vi "GUI Init - DIM.vi"(8 "error in (no error)":errorcluster, 9 "Ch.names":string[](array[string]), 10 "Cluster":T1, 11 "Array Ref.":refnum<vi>) -> (0 "error out":errorcluster, 2 "Data":dbl[](array[numeric]), 3 "Array Ref. out":refnum<vi>)   [LabVIEW 2017]
doc: "Initialize array's size and values for DIM Array by reference"
uses:
  Controls/Discrete_GUI_Cluster.ctl
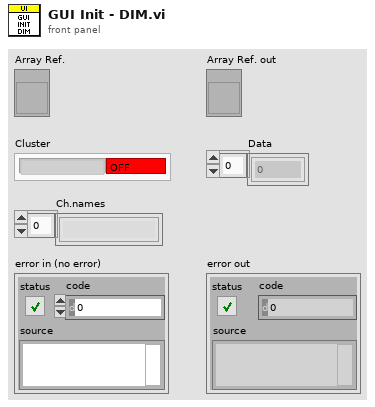
[diagram p1: front panel]
types:
  T1 = typedef "Discrete_GUI_Cluster.ctl" = cluster{"Ch.name":string, "Ch.state":bool}
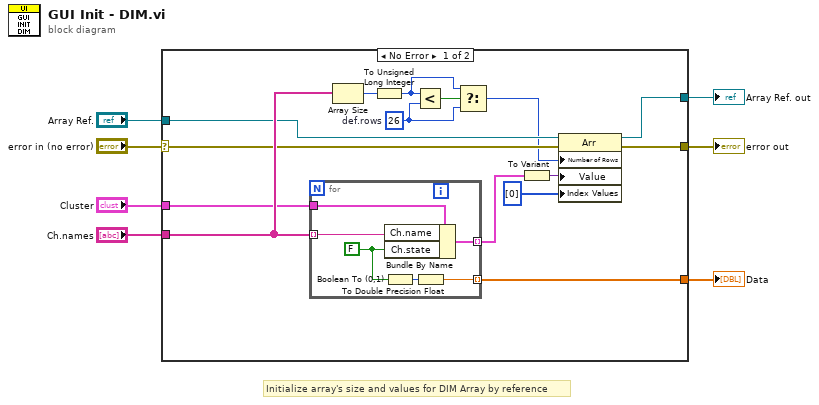
[diagram p0: block diagram]
diagram:
  # "Initialize array's size and values for DIM Array by reference"
  n1 = case shown="No Error" "error in (no error)" {
    selector: "error in (no error)" -> [w17 w30]
    tunnel: [w16 w30] -> w6
    tunnel: "Ch.names" -> [w20 _]
    tunnel: "Array Ref." -> [w19 w29]
    tunnel: "Cluster" -> [w18 _]
    tunnel: [w15 _] -> w2
    tunnel: [w12 w29] -> w1
    frame No Error {
      w10 = u32 26  # def.rows
      n2 = for {
        tunnel: [w28] -> w14 mode=indexing
        tunnel: w20 -> [w27] mode=indexing
        tunnel: w18 -> [w26]
        tunnel: [w23] -> w15 mode=indexing
        w24 = FALSE
        n3 = Bundle By Name(cluster=w26, "Ch.name"=w27, "Ch.state"=w24) -> (w28:T1)
        n4 = Boolean To (0,1)(Boolean=w24) -> (0, 1=w25:i16)
        n5 = To Double Precision Float(number=w25) -> (double precision float=w23:dbl)
      }
      n6 = Array Size(array=w20) -> (size(s)=w21:i32)
      n7 = To Unsigned Long Integer(number=w21) -> (unsigned 32bit integer=w9:u32)
      n8 = Less?(x=w9, y=w10) -> (x < y?=w11:bool)
      n9 = Select(t=w9, s=w11, f=w10) -> (s? t:f=w8:u32)
      n10 = To Variant(anything=w14) -> (Variant=w13:variant)
      n11 = property class="Arr"(reference=w19, error in=w17, "Number of Rows"=w8, "Value"=w13, "Index Values"=u32[] [0]) -> (reference out=w12:refnum<vi>, error out=w16:errorcluster)
    }
    frame Error {
    }
  }
  "error out" <- w6
  "Data" <- w2
  "Array Ref. out" <- w1
